vi "FrameCluster (SubVI).vi"(8 "y offset":dbl, 9 "x offset":dbl, 10 "index (row)":i32, 11 "ItemNames":string[][](array[string])) -> (2 "Size (m)":cluster{"Width":sgl, "Height":sgl}, 3 "Center coordinates (m)":cluster{"Xc":sgl, "Yc":sgl})   [LabVIEW 2014]
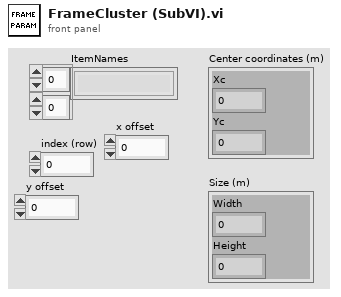
[diagram p1: front panel]
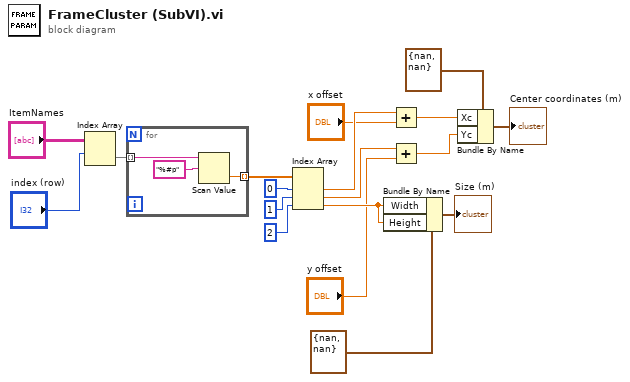
[diagram p0: block diagram]
diagram:
  n1 = Index Array(array="ItemNames", index (row)="index (row)") -> (element=w7:string[])  [unwired: 1 in]
  n2 = for {
    tunnel: w7 -> [w20] mode=indexing
    tunnel: [w19] -> w8 mode=indexing
    n3 = Scan Value(string=w20, format string="%#p") -> (value=w19:dbl)  [unwired: 1 in, 1 out]
  }
  n4 = Index Array(array=w8, index #1=0 ("index"), index #2=1 ("index"), index #3=2 ("index")) -> (element #1=w13:dbl, element #2=w14:dbl, element #3=w12:dbl)
  n5 = Bundle By Name(cluster=cluster{"Width":sgl, "Height":sgl} {"Width"=nan, "Height"=nan} ("Size (m)"), "Width"=w12, "Height"=w12) -> (→"Size (m)":cluster{"Width":sgl, "Height":sgl})
  n6 = Add(x=w13, y="x offset") -> (x+y=w4:dbl)
  n7 = Add(x=w14, y="y offset") -> (x+y=w3:dbl)
  n8 = Bundle By Name(cluster=cluster{"Xc":sgl, "Yc":sgl} {"Xc"=nan, "Yc"=nan} ("Center coordinates (m)"), "Xc"=w4, "Yc"=w3) -> (→"Center coordinates (m)":cluster{"Xc":sgl, "Yc":sgl})
